vi "download-folders-w-content.vi"(8 "error in":errorcluster, 9 "download folder":path, 10 "relative uri":string, 11 "session handle in":T1) -> (0 "error out":errorcluster, 3 "session handle out":T1)   [LabVIEW 2020]
uses:
  <vilib>/WebDAVClient/Advanced/SessionHandle.ctl
  <vilib>/WebDAVClient/NI_WebDAV.lvlib
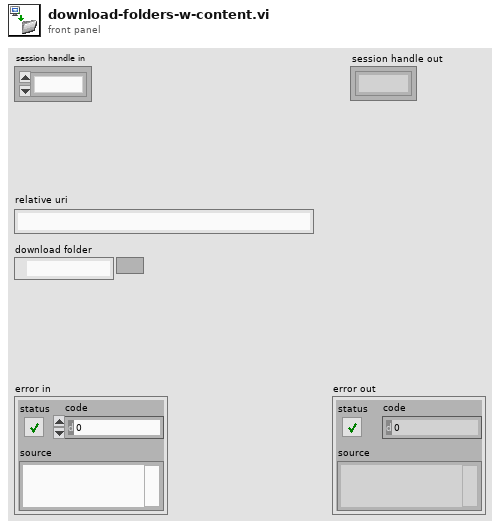
[diagram p1: front panel]
types:
  T1 = typedef "NI_WebDAV.lvlib/SessionHandle.ctl" = refnum<k1>
  T2 = typedef "NI_WebDAV.lvlib/FileInfo.ctl" = cluster{"type":string, "size":u64, "last modification":timestamp, "display name":string, "uri":string}
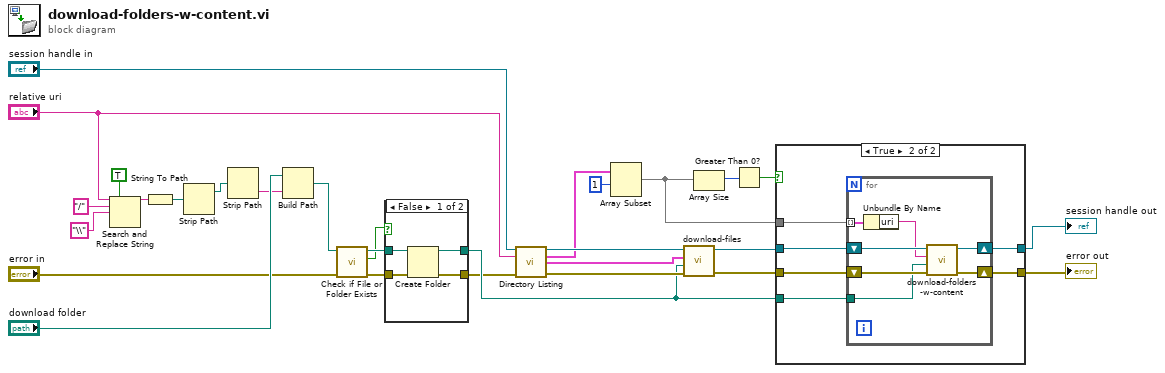
[diagram p0: block diagram]
diagram:
  n1 = Search and Replace String(replace all?=TRUE ("replace all? (F)"), input string="relative uri", search string="/", replace string="\\" ("replace string (\"\")")) -> (result string=w15:string)  [unwired: 4 in, 3 out]
  n2 = String To Path(string=w15) -> (path=w16:path)
  n3 = Strip Path(path=w16) -> (stripped path=w11:path)  [unwired: 1 out]
  n4 = Strip Path(path=w11) -> (name=w8:string)  [unwired: 1 out]
  n5 = Build Path(base path="download folder", name or relative path=w8) -> (appended path=w1:path)
  n6 = call <vilib>:"Check if File or Folder Exists.vi"("error in (no error)"="error in", "path"=w1) -> ("error out"=w5:errorcluster, "file or folder exists?"=w6:bool, "dup path"=w7:path)  [unwired: 7 in]
  n7 = case shown="False" w6 {
    tunnel: w7 -> [w33 w34]
    tunnel: w5 -> [w32 w35]
    tunnel: [w31 w35] -> w3
    tunnel: [w30 w34] -> w4
    frame False {
      n8 = Create Folder(path (use dialog)=w33, error in=w32) -> (created path=w30:path, error out=w31:errorcluster)  [unwired: 1 in, 1 out]
    }
    frame True {
    }
  }
  n9 = call <vilib>:"Directory Listing.vi"("session handle"="session handle in", "relative uri"="relative uri", "error in (no error)"=w3) -> ("session handle out"=w28:T1, "directory list"=w19:T2[], "file list"=w27:T2[], "error out"=w26:errorcluster)  [unwired: 9 in]
  n10 = Array Subset(array=w19, index=1) -> (w18:T2[])  [unwired: 1 in]
  n11 = call "download-files.vi"("error in"=w26, "download folder"=w4, "file list"=w27, "session handle in"=w28) -> ("error cout"=w23:errorcluster, "session handle out"=w21:T1)  [unwired: 6 in]
  n12 = Array Size(array=w18) -> (size(s)=w25:i32)
  n13 = Greater Than 0?(x=w25) -> (x > 0?=w24:bool)
  n14 = case shown="True" w24 {
    tunnel: w21 -> [w36 w43]
    tunnel: w23 -> [w37 w42]
    tunnel: w18 -> [_ w41]
    tunnel: w4 -> [_ w40]
    tunnel: [w37 w39] -> w22
    tunnel: [w36 w38] -> w20
    frame False {
    }
    frame True {
      n15 = for {
        tunnel: w41 -> [w47] mode=indexing
        tunnel: w40 -> [w48]
        shift-right: [w45] -> w39
        shift-left: w42 -> [w49]
        shift-right: [w44] -> w38
        shift-left: w43 -> [w50]
        n16 = Unbundle By Name(w47) -> ("uri"=w46:string)
        n17 = call "download-folders-w-content.vi"("error in"=w49, "download folder"=w48, "relative uri"=w46, "session handle in"=w50) -> ("error out"=w45:errorcluster, "session handle out"=w44:T1)  [unwired: 6 in]
      }
    }
  }
  "error out" <- w22
  "session handle out" <- w20
